vi "MicronService.vi"() -> ()   [LabVIEW 2019]
doc: "TCP Server Example. After running this VI, run the Client Write or Write Read Example."
uses:
  <vilib>/SLL Toolkit/SLL Easy TCP/_SubVIs/TCP Initialize Server - Local.vi
  <vilib>/SLL Toolkit/SLL Easy TCP/SLL Easy API via TCP.lvclass
  <vilib>/SLL Toolkit/SLL String/SLL String.lvlib
panel:
  out "Last Command Time":string
  out "Service Name":string
  out "error out":errorcluster
  out "Last Command":string
  in  "Exit":bool
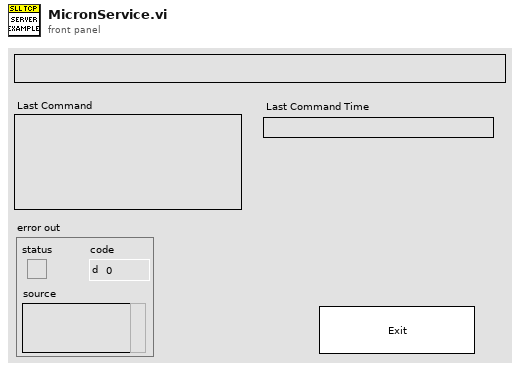
[diagram p1: front panel]
types:
  T1 = enum32{"Invalid", "Standard", "Closed", "Hidden", "Minimized", "Maximized"}
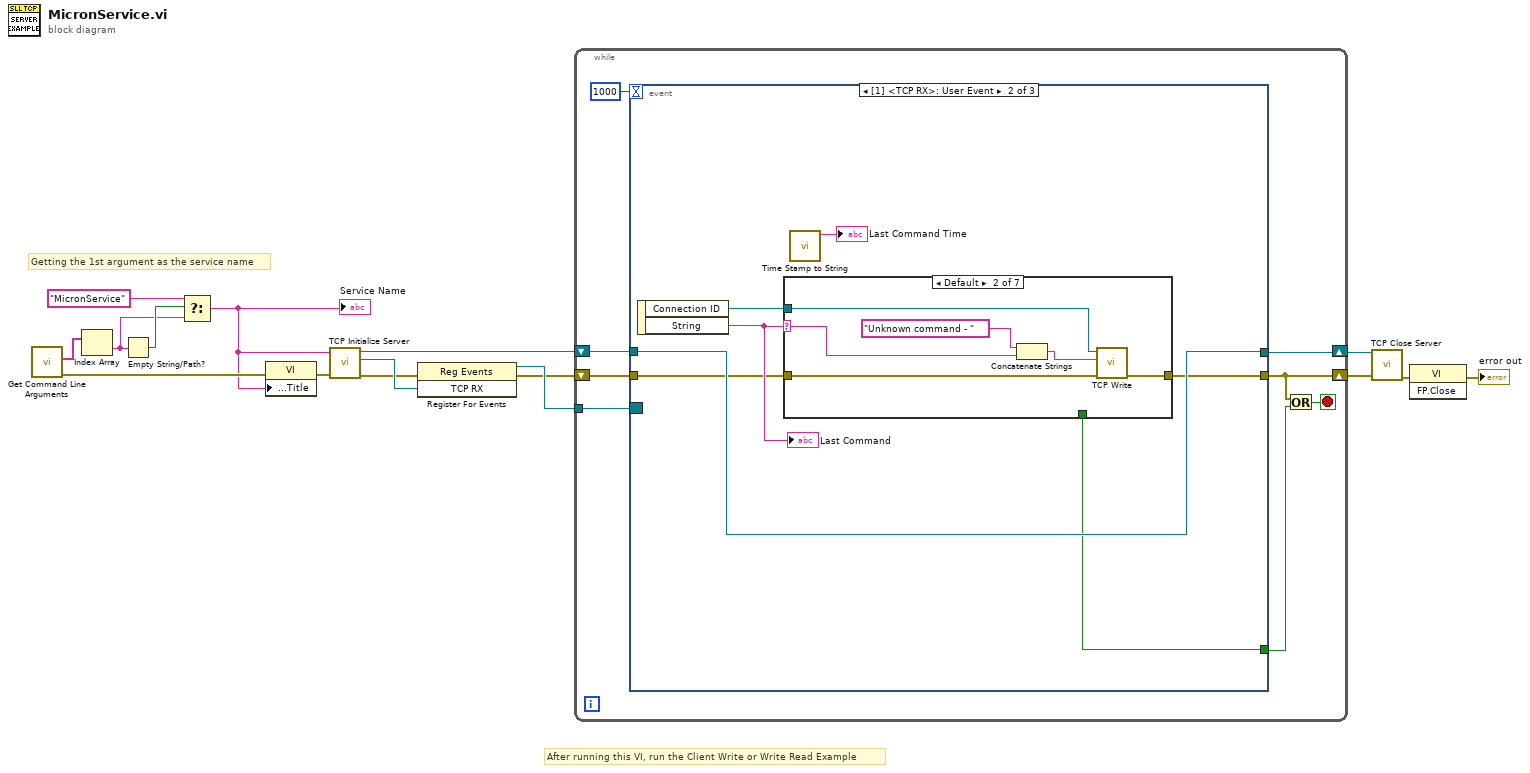
[diagram p0: block diagram]
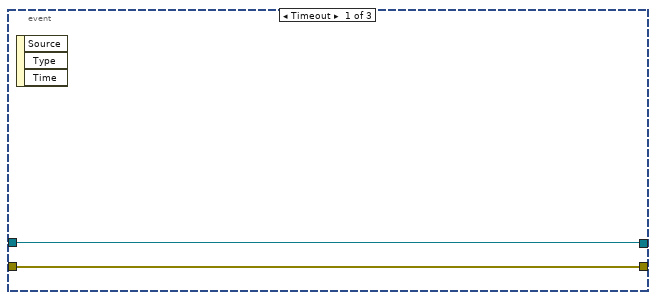
[diagram p2: hidden frame]
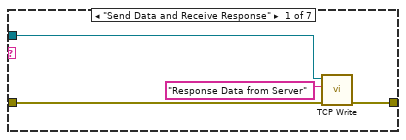
[diagram p3: hidden frame]
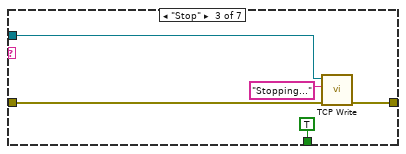
[diagram p4: hidden frame]
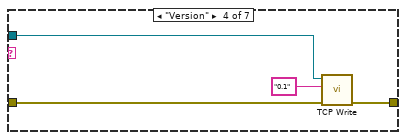
[diagram p5: hidden frame]
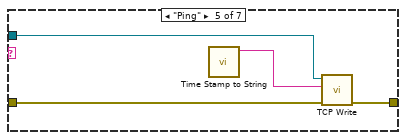
[diagram p6: hidden frame]
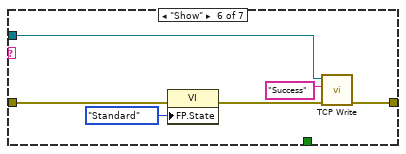
[diagram p7: hidden frame]
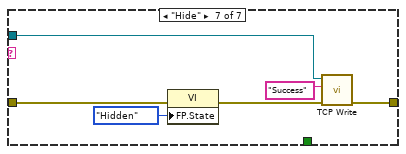
[diagram p8: hidden frame]
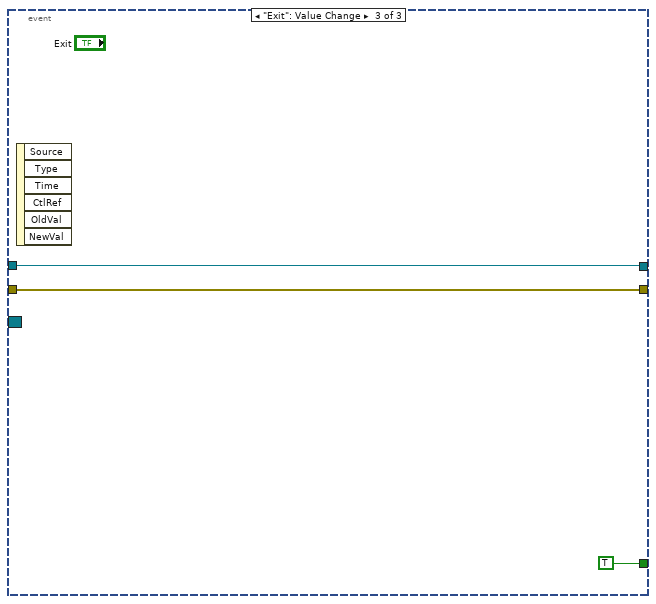
[diagram p9: hidden frame]
diagram:
  # "Getting the 1st argument as the service name"
  # "After running this VI, run the Client Write or Write Read Example"
  n1 = call <vilib>:"Get Command Line Arguments.vi"() -> ("error out"=w9:errorcluster, "arguments"=w8:string[])  [unwired: 9 in, 1 out]
  n2 = Index Array(array=w8) -> (element=w6:string)  [unwired: 1 in]
  n3 = Empty String/Path?(string/path=w6) -> (empty?=w7:bool)
  n4 = Select(t="MicronService", s=w7, f=w6) -> (s? t:f=w1:string)
  "Service Name" <- w1
  n5 = property class="VI"(error in=w9, "Front Panel.Title"=w1) -> (error out=w2:errorcluster)  [unwired: 1 in, 1 out]
  n6 = call-poly <vilib>:"TCP Initialize Server.vi"("error in (no error)"=w2, "Service Name"=w1) -> ("error out"=w12:errorcluster, "TCP RX"=w15:refnum<user-event>, "SLL Easy API via TCP out"=w16:refnum<class "SLL Easy API via TCP.lvclass">)  [unwired: 7 in]
  n7 = register-events(error in=w12, w15) -> (reference out=w14:refnum<event-registration>, error out=w11:errorcluster)  [unwired: 1 in]
  n8 = while {
    tunnel: w14 -> [w24]
    shift-right: [w19] -> w10
    shift-left: w11 -> [w20]
    shift-right: [w22] -> w13
    shift-left: w16 -> [w21]
    stop <- w17 stop-if-true
    n9 = event shown="[1] <TCP RX>: User Event" {
      selector: w24 -> [_ _ _]
      dyn-events: _ -> [_ _ _]
      timeout: 1000 -> [_ _ _]
      tunnel: [w26 w33 w71] -> w22
      tunnel: w21 -> [w26 w33 w71]
      tunnel: [_ w28 TRUE] -> w18
      tunnel: w20 -> [w25 w30 w69]
      tunnel: [w25 w29 w69] -> w19
      event Timeout {
        n10 = event-data() -> ()  [unwired: 1 in, 3 out]
      }
      event User Event {
        n11 = event-data() -> ("Connection ID"=w31:refnum<k5>, "String"=w32:string)  [unwired: 1 in]
        "Last Command" <- w32
        n12 = case shown="Default" w32 {
          selector: w32 -> [_ w39 _ _ _ _ _]
          tunnel: w31 -> [w37 w43 w48 w52 w56 w62 w68]
          tunnel: w30 -> [w35 w42 w46 w50 w55 w60 w66]
          tunnel: [w34 w41 w45 w49 w54 w59 w65] -> w29
          tunnel: [_ _ TRUE _ _ _ _] -> w28
          frame "Send Data and Receive Response" {
            n13 = call <vilib>:"TCP Write.vi"("error in (no error)"=w35, "Write Data"="Response Data from Server", "connection ID In"=w37) -> ("error out"=w34:errorcluster)  [unwired: 7 in, 1 out]
          }
          frame Default {
            n14 = Concatenate Strings("Unknown command - " ("Write Data"), w39) -> (w38:string)
            n15 = call <vilib>:"TCP Write.vi"("error in (no error)"=w42, "Write Data"=w38, "connection ID In"=w43) -> ("error out"=w41:errorcluster)  [unwired: 7 in, 1 out]
          }
          frame "Stop" {
            n16 = call <vilib>:"TCP Write.vi"("error in (no error)"=w46, "Write Data"="Stopping...", "connection ID In"=w48) -> ("error out"=w45:errorcluster)  [unwired: 7 in, 1 out]
          }
          frame "Version" {
            n17 = call <vilib>:"TCP Write.vi"("error in (no error)"=w50, "Write Data"="0.1", "connection ID In"=w52) -> ("error out"=w49:errorcluster)  [unwired: 7 in, 1 out]
          }
          frame "Ping" {
            n18 = call <vilib>:"Time Stamp to String.vi"() -> ("Output String"=w53:string)  [unwired: 11 in]
            n19 = call <vilib>:"TCP Write.vi"("error in (no error)"=w55, "Write Data"=w53, "connection ID In"=w56) -> ("error out"=w54:errorcluster)  [unwired: 7 in, 1 out]
          }
          frame "Show" {
            n20 = property class="VI"(error in=w60, "FP.State"=T1."Standard" ("Front Panel Window:State")) -> (error out=w58:errorcluster)  [unwired: 1 in, 1 out]
            n21 = call <vilib>:"TCP Write.vi"("error in (no error)"=w58, "Write Data"="Success", "connection ID In"=w62) -> ("error out"=w59:errorcluster)  [unwired: 7 in, 1 out]
          }
          frame "Hide" {
            n22 = property class="VI"(error in=w66, "FP.State"=T1."Hidden" ("Front Panel Window:State")) -> (error out=w64:errorcluster)  [unwired: 1 in, 1 out]
            n23 = call <vilib>:"TCP Write.vi"("error in (no error)"=w64, "Write Data"="Success", "connection ID In"=w68) -> ("error out"=w65:errorcluster)  [unwired: 7 in, 1 out]
          }
        }
        n24 = call <vilib>:"Time Stamp to String.vi"() -> ("Output String"=→"Last Command Time":string)  [unwired: 11 in]
      }
      event "Exit": Value Change {
        n25 = event-data() -> ()  [unwired: 1 in, 6 out]
      }
    }
    n26 = Or(x=w19, y=w18) -> (x .or. y?=w17:bool)
  }
  n27 = call <vilib>:"TCP Close Server.vi"("error in (no error)"=w10, "SLL Easy API via TCP in"=w13) -> ("error out"=w4:errorcluster)  [unwired: 9 in]
  n28 = invoke class="VI" method="FP.Close"(error in=w4) -> (error out=→"error out":errorcluster)  [unwired: 2 in, 2 out]
